vi "Encoder Quad Phase Detection.vi"(8 "Phase B":bool, 9 "Phase A":bool, 10 "Clear Error?":bool, 11 "Enable?":bool) -> (1 "Signal":bool, 2 "Backward?":bool, 3 "Error":bool)   [LabVIEW 2015]
uses:
  Encoder States.ctl
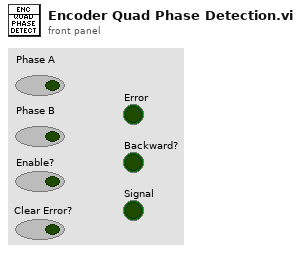
[diagram p1: front panel]
types:
  T1 = typedef "Encoder States.ctl" = fxp<+,3,3>
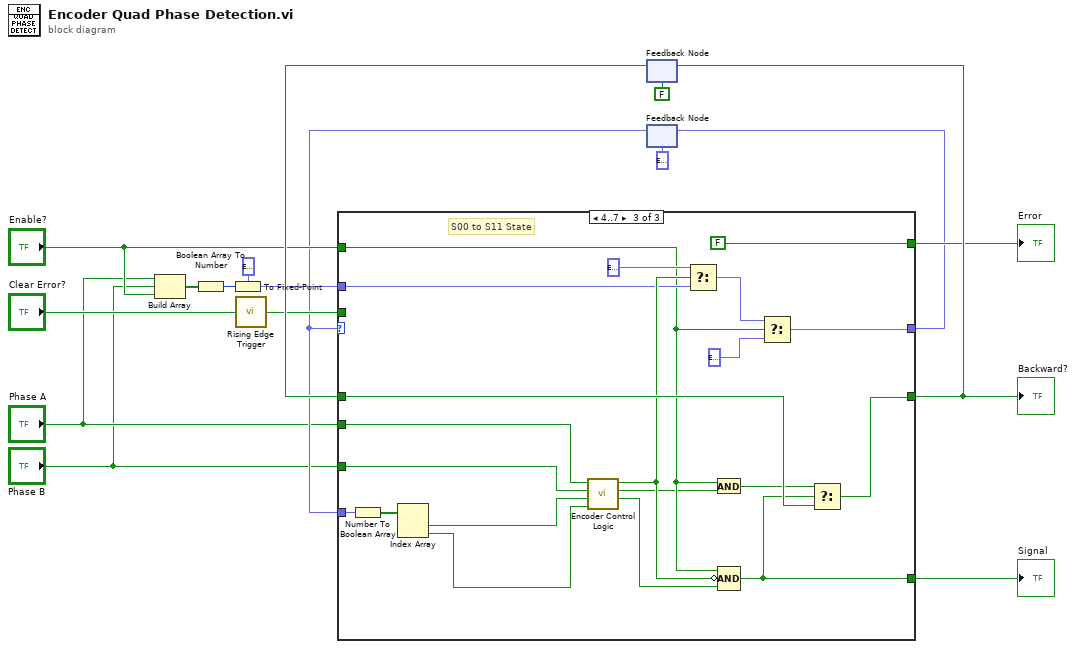
[diagram p0: block diagram]
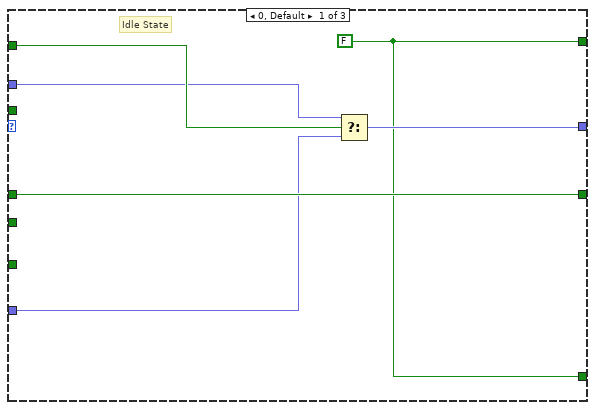
[diagram p2: hidden frame]
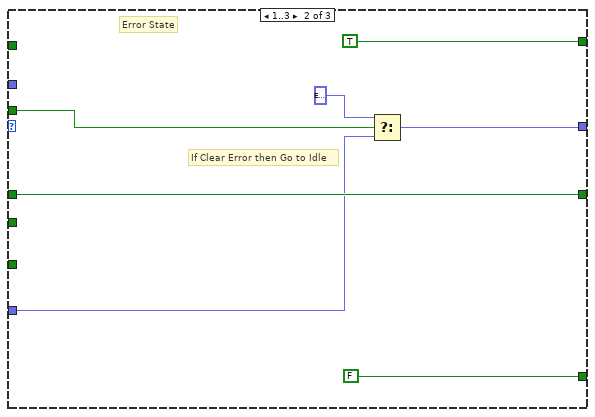
[diagram p3: hidden frame]
diagram:
  n1 = Build Array("Phase A", "Phase B", "Enable?") -> (w6:bool[])
  n2 = Boolean Array To Number(Boolean array=w6) -> (number=w5:u8)
  n3 = To Fixed-Point(fixed-point type=T1 0.0 ("Numeric"), number=w5) -> (fixed-point=w3:T1)
  n4 = call "Rising Edge Trigger.vi"("Signal"="Clear Error?") -> ("Trigger?"=w9:bool)
  n5 = feedback #1(FALSE ("Direction")) -> (w11:bool)
  n6 = feedback #2(T1 0.0) -> (w7:T1)
  n7 = case shown="4..7" w7 {
    tunnel: "Enable?" -> [w23 _ w37]
    tunnel: [w21 w27 w41] -> w13
    tunnel: [w19 TRUE ("Error") FALSE ("Error")] -> w15
    tunnel: w3 -> [w22 _ w45]
    tunnel: w11 -> [w20 w29 w50]
    tunnel: [w20 w29 w49] -> w16
    tunnel: [w19 FALSE ("Error") w39] -> w17
    tunnel: w9 -> [_ w28 _]
    tunnel: "Phase B" -> [_ _ w47]
    tunnel: "Phase A" -> [_ _ w48]
    tunnel: w7 -> [w18 w24 w32]
    frame 0, Default {
      w19 = FALSE ("Error")
      # "Idle State"
      n8 = Select(t=w22, s=w23, f=w18) -> (s? t:f=w21:T1)
    }
    frame 1..3 {
      # "Error State"
      # "If Clear Error then Go to Idle"
      n9 = Select(t=T1 0.0, s=w28, f=w24) -> (s? t:f=w27:T1)
    }
    frame 4..7 {
      # "S00 to S11 State"
      n10 = Number To Boolean Array(number=w32) -> (Boolean array=w34:bool[])
      n11 = Index Array(array=w34) -> (element #1=w33:bool, element #2=w31:bool)  [unwired: 2 in]
      n12 = call "Encoder Control Logic.vi"("Prev Phase B (State Bit 1)"=w31, "Prev Phase A (State Bit 0)"=w33, "Phase B"=w47, "Phase A"=w48) -> ("Count?"=w36:bool, "Backward?"=w35:bool, "Error Occurred?"=w46:bool)  [unwired: 5 in]
      n13 = Select(t=T1 1.0, s=w46, f=w45) -> (s? t:f=w43:T1)
      n14 = And(x=w37, y=w35) -> (x .and. y?=w38:bool)
      n15 = Compound Arithmetic op=AND(w37, invert w46, w36) -> (w39:bool)
      n16 = Select(t=w43, s=w37, f=T1 0.0) -> (s? t:f=w41:T1)
      n17 = Select(t=w38, s=w39, f=w50) -> (s? t:f=w49:bool)
    }
  }
  "Backward?" <- w16
  "Signal" <- w17
  "Error" <- w15
  n18 = feedback-in #1(w16) -> ()
  n19 = feedback-in #2(w13) -> ()
